vi "init.vi"(8 "error in":errorcluster, 11 "Param in":refnum<class "TCP Param.lvclass">) -> (0 "error":errorcluster, 3 "Param out":refnum<class "TCP Param.lvclass">)   [LabVIEW 2021, in "Param.lvlib" / "TCP Param.lvclass"]
uses:
  TCP Param.lvclass
  Typedefs/timeouts.ctl
  TCP Param.lvclass/TCP Param.ctl
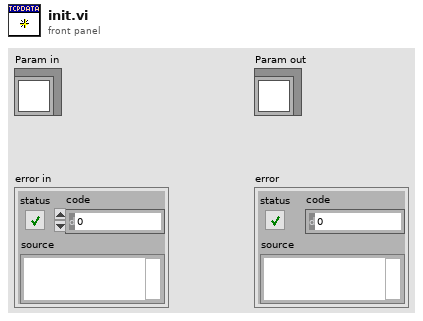
[diagram p1: front panel]
types:
  T1 = typedef "Param.lvlib/TCP Param.lvclass/timeouts.ctl" = cluster{"conn_timeout":i32, "reconn_timeout":i32, "N attempt max":i32, "t_reset_TTL":i32, "write_timeout":i32, "read_timeout":i32, "period":i32}
  T2 = cluster{"IP address":cluster{"Remote IP Address":string, "Remote Port":u16}, "timeouts":T1}
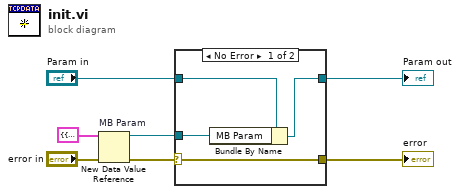
[diagram p0: block diagram]
diagram:
  n1 = New Data Value Reference "MB Param"(data value=T2 {"IP address"={"Remote IP Address"="", "Remote Port"=0}, "timeouts"={"conn_timeout"=0, "reconn_timeout"=0, "N attempt max"=0, "t_reset_TTL"=0, "write_timeout"=0, "read_timeout"=0, "period"=0}} ("MB Param"), error in="error in") -> (data value reference=w7:refnum<data-value>, error out=w2:errorcluster)
  n2 = case shown="No Error" w2 {
    selector: w2 -> [w11 w13]
    tunnel: w7 -> [w9 _]
    tunnel: [w11 w13] -> w5
    tunnel: "Param in" -> [w10 w12]
    tunnel: [w8 w12] -> w1
    frame No Error {
      n3 = Bundle By Name(cluster=w10, "MB Param"=w9) -> (w8:refnum<class "TCP Param.lvclass">)
    }
    frame Error {
    }
  }
  "error" <- w5
  "Param out" <- w1
